vi "MecaOdometry_UpdateWithTime.vi"(8 "WheelSpeeds":T7 {"RearRightSpeed" format="%19.3f"; "RearLeftSpeed" format="%19.3f"; "FrontRightSpeed" format="%19.3f"; "FrontLeftSpeed" format="%19.3f"}, 9 "GyroAngle":T4={"VALUE"=0.0, "COS"=1.0, "SIN"=0.0} {"SIN" format="%13.4f"; "COS" format="%13.4f"; "VALUE" format="%13.4f"}, 10 "CurrentTime":dbl format="%24.4f", 11 "in MECA_DRIVE_ODOMETRY":T1={"POSE"={"TRANSLATION"={"X"=0.0, "Y"=0.0}, "ROTATION"={"VALUE"=0.0, "COS"=1.0, "SIN"=0.0}}, "PrevTime"=0.0, "GyroOffset"={"VALUE"=0.0, "COS"=0.0, "SIN"=0.0}, "PreviousAngle"={"VALUE"=0.0, "COS"=0.0, "SIN"=0.0}, "Kinematics"={"FrontLeft"={"X"=0.0, "Y"=0.0}, "FrontRight"={"X"=0.0, "Y"=0.0}, "RearLeft"={"X"=0.0, "Y"=0.0}, "RearRight"={"X"=0.0, "Y"=0.0}, "InverseKinematics"=[[0.0, 1.0, -1.0, 0.0], [0.0, 1.0, 1.0, 0.0], [0.0, 1.0, 1.0, 0.0], [0.0, 1.0, -1.0, 0.0]], "ForwardKinematics"=[[0.0, 1.0, -1.0, 0.0], [0.0, 1.0, 1.0, 0.0], [0.0, 1.0, 1.0, 0.0], [0.0, 1.0, -1.0, 0.0]], "PrevCoR"={"X"=0.0, "Y"=0.0}}} {"Kinematics"."PrevCoR"."Y" format="%14.3f"; "Kinematics"."PrevCoR"."X" format="%14.3f"; "Kinematics"."RearRight"."Y" format="%14.3f"; "Kinematics"."RearRight"."X" format="%14.3f"; "Kinematics"."RearLeft"."Y" format="%14.3f"; "Kinematics"."RearLeft"."X" format="%14.3f"; "Kinematics"."FrontRight"."Y" format="%14.3f"; "Kinematics"."FrontRight"."X" format="%14.3f"; "Kinematics"."FrontLeft"."Y" format="%14.3f"; "Kinematics"."FrontLeft"."X" format="%14.3f"; "PreviousAngle"."SIN" format="%13.4f"; "PreviousAngle"."COS" format="%13.4f"; "PreviousAngle"."VALUE" format="%13.4f"; "GyroOffset"."SIN" format="%13.4f"; "GyroOffset"."COS" format="%13.4f"; "GyroOffset"."VALUE" format="%13.4f"; "PrevTime" format="%13.4f"; "POSE"."ROTATION"."SIN" format="%13.4f"; "POSE"."ROTATION"."COS" format="%13.4f"; "POSE"."ROTATION"."VALUE" format="%13.4f"; "POSE"."TRANSLATION"."Y" format="%14.3f"; "POSE"."TRANSLATION"."X" format="%14.3f"}) -> (1 "POSE":T2={"TRANSLATION"={"X"=0.0, "Y"=0.0}, "ROTATION"={"VALUE"=0.0, "COS"=1.0, "SIN"=0.0}} {"ROTATION"."SIN" format="%13.4f"; "ROTATION"."COS" format="%13.4f"; "ROTATION"."VALUE" format="%13.4f"; "TRANSLATION"."Y" format="%14.3f"; "TRANSLATION"."X" format="%14.3f"}, 3 "out MECA_DRIVE_ODOMETRY":T1={"POSE"={"TRANSLATION"={"X"=0.0, "Y"=0.0}, "ROTATION"={"VALUE"=0.0, "COS"=1.0, "SIN"=0.0}}, "PrevTime"=0.0, "GyroOffset"={"VALUE"=0.0, "COS"=0.0, "SIN"=0.0}, "PreviousAngle"={"VALUE"=0.0, "COS"=0.0, "SIN"=0.0}, "Kinematics"={"FrontLeft"={"X"=0.0, "Y"=0.0}, "FrontRight"={"X"=0.0, "Y"=0.0}, "RearLeft"={"X"=0.0, "Y"=0.0}, "RearRight"={"X"=0.0, "Y"=0.0}, "InverseKinematics"=[[0.0, 1.0, -1.0, 0.0], [0.0, 1.0, 1.0, 0.0], [0.0, 1.0, 1.0, 0.0], [0.0, 1.0, -1.0, 0.0]], "ForwardKinematics"=[[0.0, 1.0, -1.0, 0.0], [0.0, 1.0, 1.0, 0.0], [0.0, 1.0, 1.0, 0.0], [0.0, 1.0, -1.0, 0.0]], "PrevCoR"={"X"=0.0, "Y"=0.0}}} {"Kinematics"."PrevCoR"."Y" format="%14.3f"; "Kinematics"."PrevCoR"."X" format="%14.3f"; "Kinematics"."RearRight"."Y" format="%14.3f"; "Kinematics"."RearRight"."X" format="%14.3f"; "Kinematics"."RearLeft"."Y" format="%14.3f"; "Kinematics"."RearLeft"."X" format="%14.3f"; "Kinematics"."FrontRight"."Y" format="%14.3f"; "Kinematics"."FrontRight"."X" format="%14.3f"; "Kinematics"."FrontLeft"."Y" format="%14.3f"; "Kinematics"."FrontLeft"."X" format="%14.3f"; "PreviousAngle"."SIN" format="%13.4f"; "PreviousAngle"."COS" format="%13.4f"; "PreviousAngle"."VALUE" format="%13.4f"; "GyroOffset"."SIN" format="%13.4f"; "GyroOffset"."COS" format="%13.4f"; "GyroOffset"."VALUE" format="%13.4f"; "PrevTime" format="%13.4f"; "POSE"."ROTATION"."SIN" format="%13.4f"; "POSE"."ROTATION"."COS" format="%13.4f"; "POSE"."ROTATION"."VALUE" format="%13.4f"; "POSE"."TRANSLATION"."Y" format="%14.3f"; "POSE"."TRANSLATION"."X" format="%14.3f"})   [LabVIEW 2019, in "Trajectory_Library.lvlib"]
doc: "Updates the robot's position on the field using forward kinematics and integration of the pose over time. This method takes in the current time as a parameter to calculate period (difference between two timestamps). The period is used to calculate the change in distance from a velocity. This also takes in an angle parameter which is used instead of the angular rate that is calculated from forward kinematics.\n \nParameters:\n - MecaDriveOdometry - Data structure\n - currentTime - The current time in seconds.\n - gyroAngle - The angle reported by the gyroscope.\n - wheelSpeeds - The current wheel speeds.\n\nReturns:\n - MecaDriveOdometry - Updated data structure\n - Pose - The new pose of the robot."
uses:
  Trajectory_Library.lvlib
  TypeDef/TRANSLATION2D.ctl
  TypeDef/ROTATION2D.ctl
  TypeDef/POSE2D.ctl
  TypeDef/MECA_DRIVE_ODOMETRY.ctl
  TypeDef/MECA_WHEEL_SPEEDS.ctl
  <vilib>/Analysis/Matrix/Datatypes/RealMatrix.ctl
  <vilib>/Analysis/Matrix/NI_Matrix.lvlib
  TypeDef/MECA_DRIVE_KINEMATICS.ctl
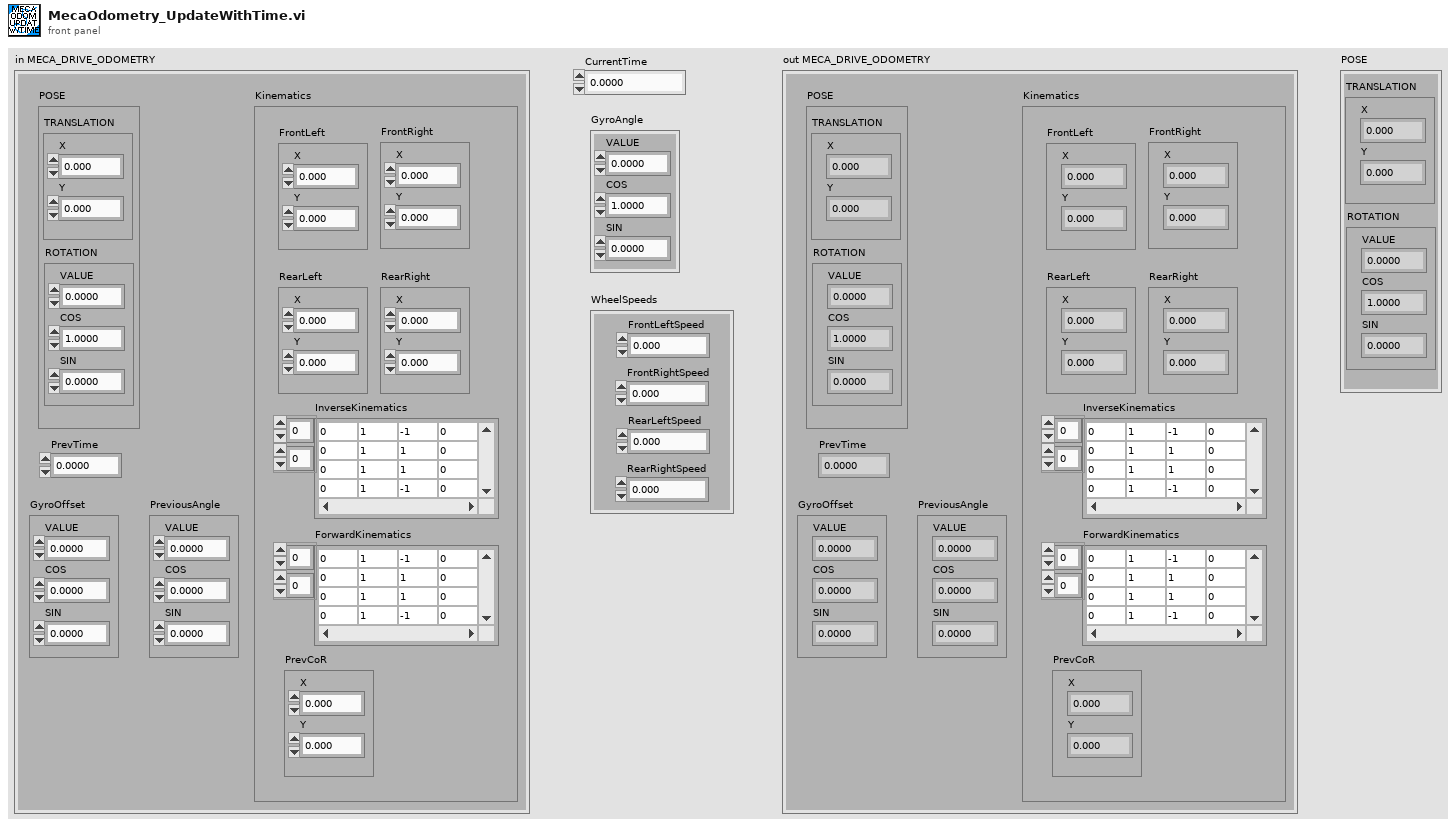
[diagram p1: front panel]
types:
  T1 = typedef "Trajectory_Library.lvlib/MECA_DRIVE_ODOMETRY.ctl" = cluster{"POSE":T2, "PrevTime":dbl, "GyroOffset":T4, "PreviousAngle":T4, "Kinematics":T5}
  T2 = typedef "Trajectory_Library.lvlib/POSE2D.ctl" = cluster{"TRANSLATION":T3, "ROTATION":T4}
  T3 = typedef "Trajectory_Library.lvlib/TRANSLATION2D.ctl" = cluster{"X":dbl, "Y":dbl}
  T4 = typedef "Trajectory_Library.lvlib/ROTATION2D.ctl" = cluster{"VALUE":dbl, "COS":dbl, "SIN":dbl}
  T5 = typedef "Trajectory_Library.lvlib/MECA_DRIVE_KINEMATICS.ctl" = cluster{"FrontLeft":T3, "FrontRight":T3, "RearLeft":T3, "RearRight":T3, "InverseKinematics":T6, "ForwardKinematics":T6, "PrevCoR":T3}
  T6 = typedef "NI_Matrix.lvlib/RealMatrix.ctl" = dbl[][]
  T7 = typedef "Trajectory_Library.lvlib/MECA_WHEEL_SPEEDS.ctl" = cluster{"FrontLeftSpeed":dbl, "FrontRightSpeed":dbl, "RearLeftSpeed":dbl, "RearRightSpeed":dbl}
  T8 = typedef "Trajectory_Library.lvlib/CHASSIS_SPEEDS.ctl" = cluster{"vX":dbl, "vY":dbl, "vOmega":dbl}
  T9 = typedef "Trajectory_Library.lvlib/TWIST2D.ctl" = cluster{"dX":dbl, "dY":dbl, "dTHETA":dbl}
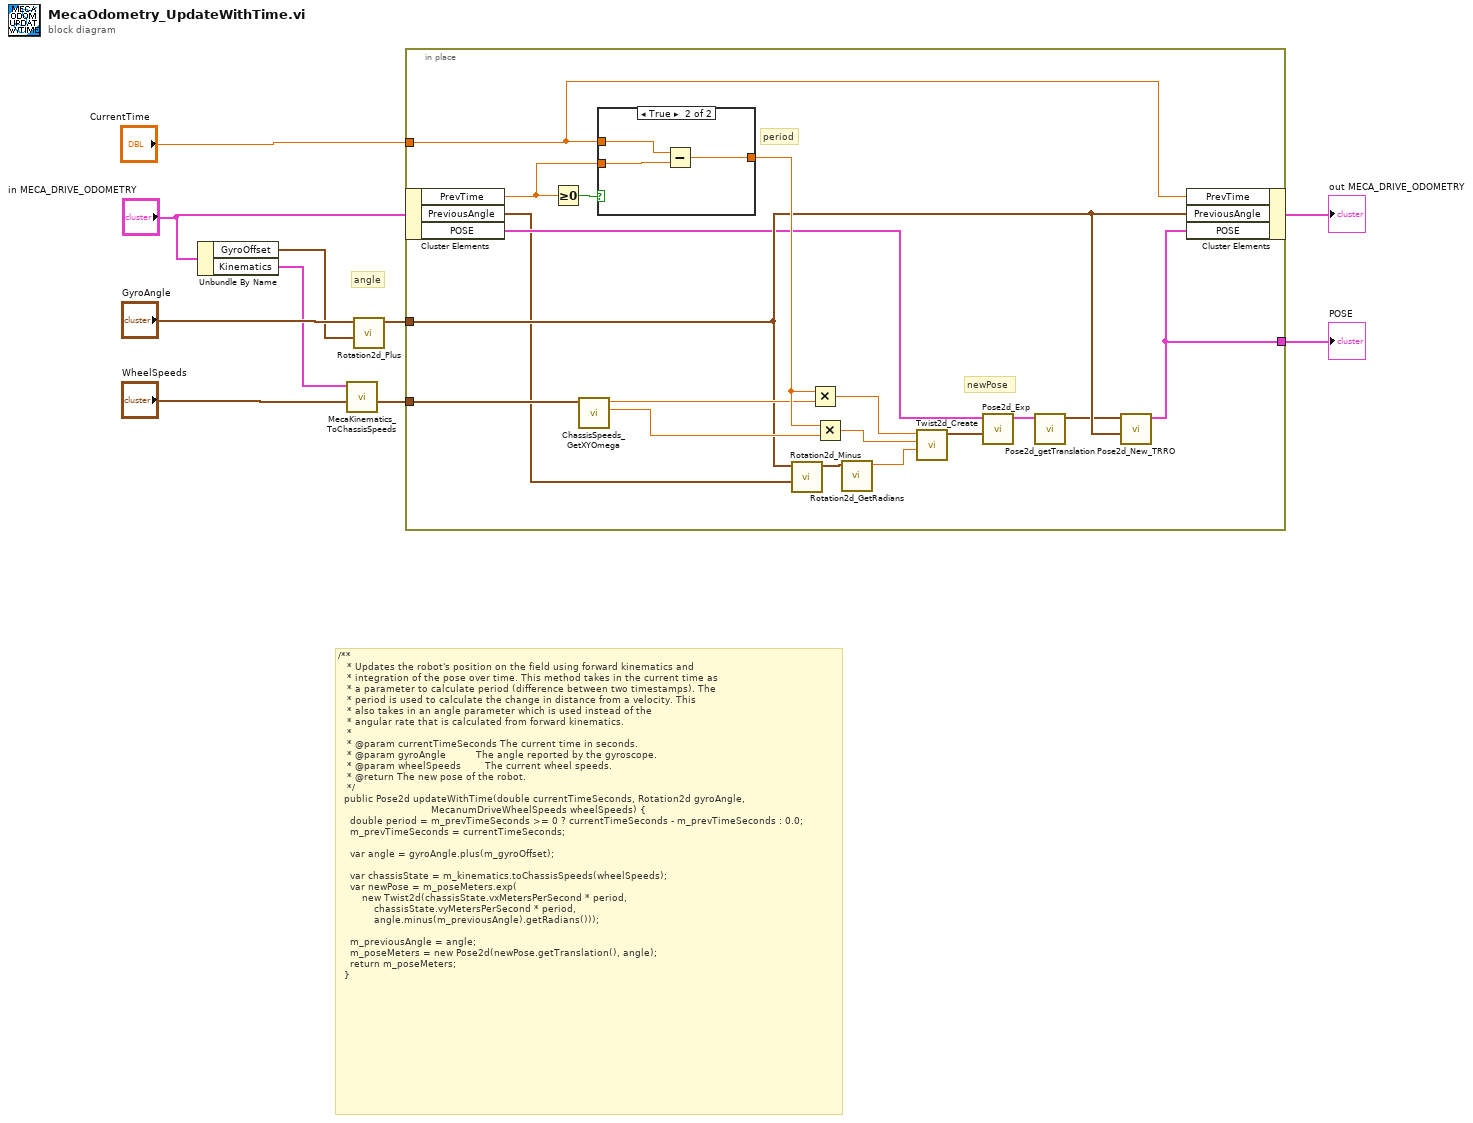
[diagram p0: block diagram]
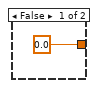
[diagram p2: hidden frame]
diagram:
  # "angle"
  # "/**\n   * Updates the robot's position on the field using forward kinematics and\n   * integration of the pose over time. This method takes in the current time as\n   * a parameter to calculate period (difference between two timestamps). The\n   * period is used to calculate the change in distance from a velocity. This\n   * also takes in an angle parameter which is used instead of the\n   * angular rate that is calculated from forward kinematics.\n   *\n   * @param currentTimeSeconds The current time in seconds.\n   * @param gyroAngle          The angle reported by the gyroscope.\n   * @param wheelSpeeds        The current wheel speeds.\n   * @return The new pose of the robot.\n   */\n  public Pose2d updateWithTime(double currentTimeSeconds, Rotation2d gyroAngle,\n                               MecanumDriveWheelSpeeds wheelSpeeds) {\n    double period = m_prevTimeSeconds >= 0 ? currentTimeSeconds - m_prevTimeSeconds : 0.0;\n    m_prevTimeSeconds = currentTimeSeconds;\n\n    var angle = gyroAngle.plus(m_gyroOffset);\n\n    var chassisState = m_kinematics.toChassisSpeeds(wheelSpeeds);\n    var newPose = m_poseMeters.exp(\n        new Twist2d(chassisState.vxMetersPerSecond * period,\n            chassisState.vyMetersPerSecond * period,\n            angle.minus(m_previousAngle).getRadians()));\n\n    m_previousAngle = angle;\n    m_poseMeters = new Pose2d(newPose.getTranslation(), angle);\n    return m_poseMeters;\n  }"
  n1 = Unbundle By Name("in MECA_DRIVE_ODOMETRY") -> ("GyroOffset"=w4:T4, "Kinematics"=w5:T5)
  n2 = call "MecaKinematics_ToChassisSpeeds.vi"("MECA_WHEEL_SPEEDS"="WheelSpeeds", "in MECA_DRIVE_KINEMATICS"=w5) -> ("ChassisSpeeds"=w3:T8)  [unwired: 9 in]
  n3 = call "Rotation2d_Plus.vi"("other ROTATION"=w4, "in ROTATION"="GyroAngle") -> ("out ROTATION"=w7:T4)  [unwired: 9 in]
  n4 = in-place {
    in-place-border: "CurrentTime" -> [w20]
    in-place-border: w7 -> [w19]
    in-place-border: [w18] -> w6
    in-place-border: w3 -> [w23]
    # "newPose"
    # "period"
    n5 = in-place-cluster #1("in MECA_DRIVE_ODOMETRY") -> ("PrevTime"=w17:dbl, "PreviousAngle"=w15:T4, "POSE"=w16:T2)
    n6 = Greater Or Equal To 0?(x=w17) -> (x >= 0?=w28:bool)
    n7 = call "ChassisSpeeds_GetXYOmega.vi"("CHASSIS"=w23) -> ("vY"=w21:dbl, "vX"=w22:dbl)  [unwired: 8 in, 1 out]
    n8 = case shown="True" w28 {
      tunnel: w20 -> [_ w32]
      tunnel: w17 -> [_ w31]
      tunnel: [0.0 w30] -> w27
      frame False {
      }
      frame True {
        n9 = Subtract(x=w32, y=w31) -> (x-y=w30:dbl)
      }
    }
    n10 = call "Rotation2d_Minus.vi"("other ROTATION"=w15, "in ROTATION"=w19) -> ("out ROTATION"=w14:T4)  [unwired: 9 in]
    n11 = Multiply(x=w27, y=w22) -> (x*y=w26:dbl)
    n12 = Multiply(x=w27, y=w21) -> (x*y=w25:dbl)
    n13 = call "Rotation2d_GetRadians.vi"("in ROTATION"=w14) -> ("AngleRadians"=w13:dbl)  [unwired: 10 in]
    n14 = call "Twist2d_Create.vi"("dTHETA"=w13, "dY"=w25, "dX"=w26) -> ("TWIST"=w24:T9)  [unwired: 8 in]
    n15 = call "Pose2d_Exp.vi"("TWIST"=w24, "POSE"=w16) -> ("UpdatedPose"=w12:T2)  [unwired: 9 in]
    n16 = call "Pose2d_getTranslation.vi"("in POSE"=w12) -> ("outTRANSLATION"=w11:T3)  [unwired: 10 in]
    n17 = call "Pose2d_New_TRRO.vi"("ROTATION"=w19, "TRANSLATION"=w11) -> ("outPOSE"=w18:T2)  [unwired: 9 in]
    n18 = in-place-cluster #1("PrevTime"=w20, "PreviousAngle"=w19, "POSE"=w18) -> (→"out MECA_DRIVE_ODOMETRY":T1)
  }
  "POSE" <- w6
